vi "Quick Permutation.vi"(11 "Array to Permutate":string[](array[string])=["0", "1", "2", "3", "4", "5", "6", "7", "8", "9"]) -> (2 "# Permutations":i32, 3 "Permutations":string[](array[string]))   [LabVIEW 2013, in "Problem 24.lvlib"]
uses:
  Problem 24.lvlib
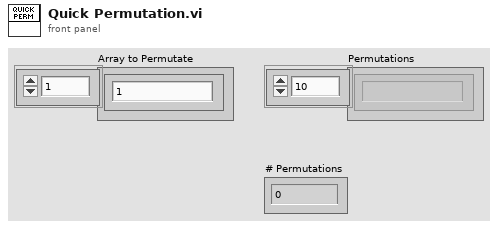
[diagram p1: front panel]
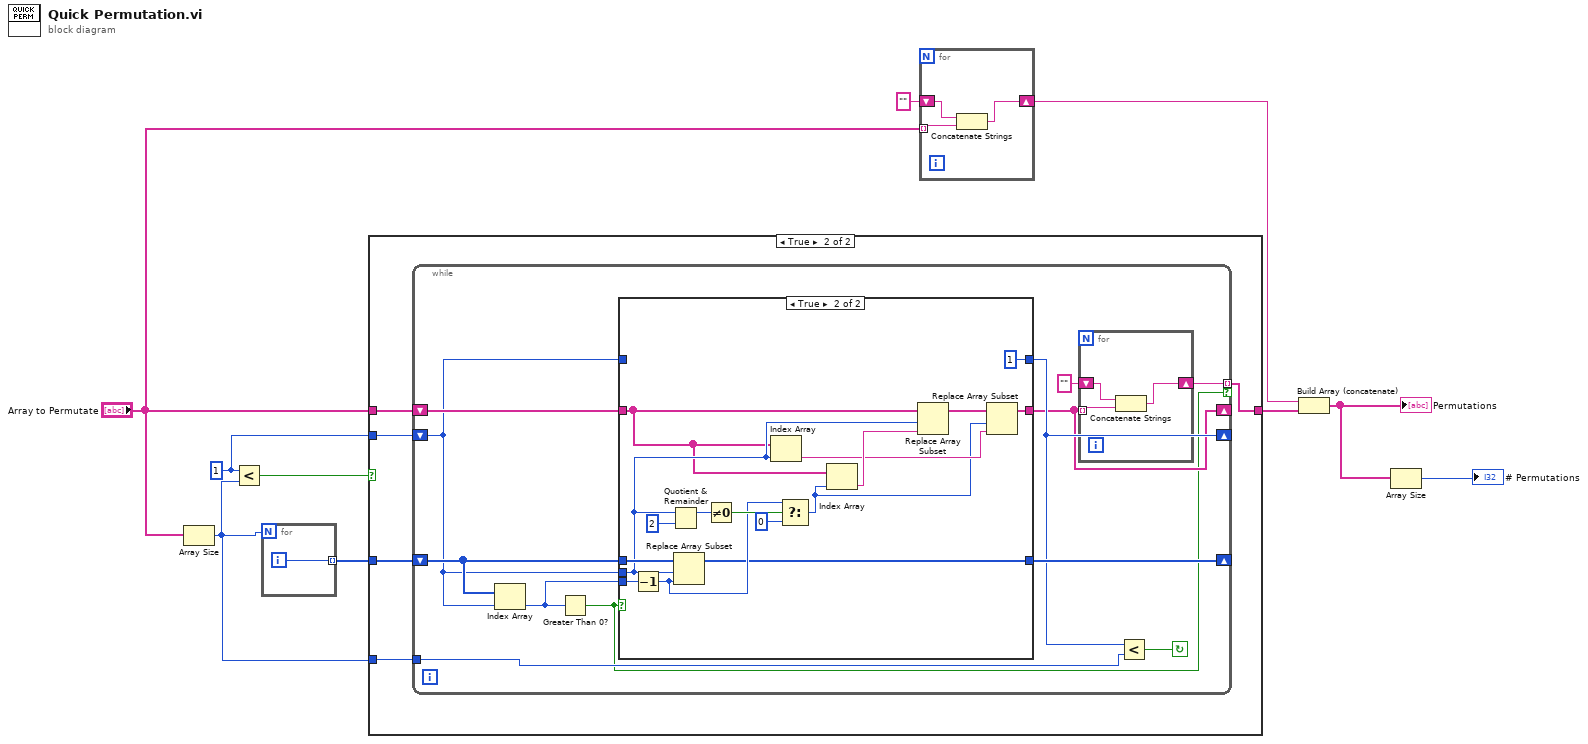
[diagram p0: block diagram]
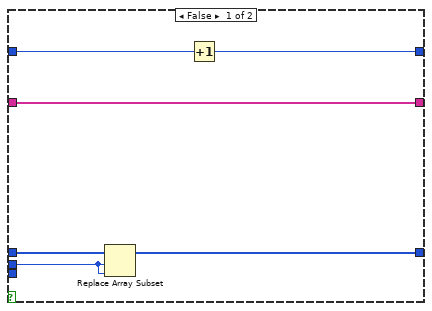
[diagram p3: hidden frame]
diagram:
  w9 = 1 ("x")
  n1 = Array Size(array="Array to Permutate") -> (size(s)=w1:i32)
  n2 = Less?(x=w9, y=w1) -> (x < y?=w8:bool)
  n3 = for {
    N: w1 -> [_]
    tunnel: [w11] -> w10 mode=indexing
    i -> [w11]
  }
  n4 = case shown="True" w8 {
    tunnel: "Array to Permutate" -> [w12 w15]
    tunnel: w9 -> [_ w17]
    tunnel: w10 -> [_ w16]
    tunnel: w1 -> [_ w14]
    tunnel: [w12 w13] -> w6
    frame False {
    }
    frame True {
      n5 = while {
        shift-right: [w22] -> _
        shift-left: w17 -> [w26]
        shift-right: [w23] -> _
        shift-left: w16 -> [w29]
        tunnel: w14 -> [w25]
        shift-right: [w19] -> _
        shift-left: w15 -> [w27]
        tunnel: [w20] -> w13 mode=indexing if=w18
        stop <- w24 continue-if-true
        n6 = Index Array(array=w29, index=w26) -> (element=w28:i32)
        n7 = Greater Than 0?(x=w28) -> (x > 0?=w18:bool)
        n8 = case shown="True" w18 {
          tunnel: w29 -> [w38 w54]
          tunnel: w26 -> [w37 w47]
          tunnel: w28 -> [_ w53]
          tunnel: w27 -> [w33 w46]
          tunnel: w26 -> [w36 _]
          tunnel: [w35 1] -> w22
          tunnel: [w34 w40] -> w23
          tunnel: [w33 w39] -> w19
          frame False {
            n9 = Replace Array Subset(array=w38, new element=w37, index=w37) -> (w34:i32[])
            n10 = Increment(x=w36) -> (x+1=w35:i32)
          }
          frame True {
            n11 = Decrement(x=w53) -> (x-1=w48:i32)
            n12 = Quotient & Remainder(x=w47, y=2) -> (x-y*floor(x/y)=w51:i32)  [unwired: 1 out]
            n13 = Replace Array Subset(array=w54, new element=w48, index=w47) -> (w40:i32[])
            n14 = Not Equal To 0?(x=w51) -> (x != 0?=w50:bool)
            n15 = Index Array(array=w46, index=w47) -> (element=w43:string)
            n16 = Select(t=w48, s=w50, f=0 ("y")) -> (s? t:f=w42:i32)
            n17 = Index Array(array=w46, index=w42) -> (element=w45:string)
            n18 = Replace Array Subset(array=w46, new element=w45, index=w47) -> (w44:string[])
            n19 = Replace Array Subset(array=w44, new element=w43, index=w42) -> (w39:string[])
          }
        }
        n20 = for {
          tunnel: w19 -> [w30] mode=indexing
          shift-right: [w31] -> w20
          shift-left: "" -> [w32]
          n21 = Concatenate Strings(w32, w30) -> (w31:string)
        }
        n22 = Less?(x=w22, y=w25) -> (x < y?=w24:bool)
      }
    }
  }
  n23 = for {
    tunnel: "Array to Permutate" -> [w56] mode=indexing
    shift-right: [w55] -> w2
    shift-left: "" -> [w57]
    n24 = Concatenate Strings(w57, w56) -> (w55:string)
  }
  n25 = Build Array (concatenate)(w2, w6) -> (w7:string[])
  "Permutations" <- w7
  n26 = Array Size(array=w7) -> (size(s)=→"# Permutations":i32)
